vi "SECoP-getStoredCommand_2.vi"(8 "error in (no error)":errorcluster, 11 "DLL path (in)":T2) -> (0 "error out":errorcluster, 1 "arguments/setvalue":string, 2 "command/parameter path":string, 3 "DLL path (out)":T2, 4 "action":T1, 5 "command id":u64)   [LabVIEW 2023, in "SECoP.lvlib"]
doc: "Call <b>\"SECoP-getStoredCommand_2.vi\"</b> regulary to check, if there is something to do for any accessible. If yes, it will return successfully with an id, what to do, a parameter/command name and new set value or argument as JSON string.\n\n<b>DLL path</b> input and output of cluster from \"SECoP-Initialize.vi\"\n<b>command id</b> on match: command id for \"SECoP-putCommandAnswer_2.vi\"\n<b>action id</b> on match: action id to handle\n<b>command/parameter path</b> on match: full name of accessible\n<b>arguments/setvalue</b> on match with change or do: JSON input data from SECoP-client"
uses:
  SECoP.lvlib
  SECoP-libraries.ctl
  SECoP-action.ctl
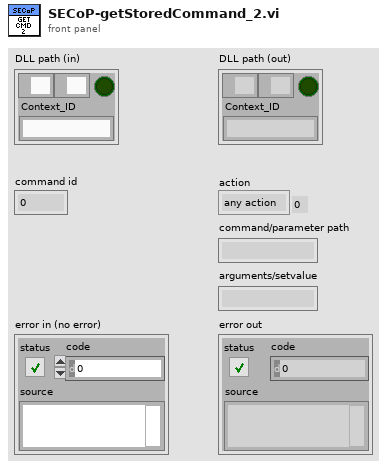
[diagram p1: front panel]
types:
  T1 = typedef "SECoP.lvlib/SECoP-action.ctl" = enum32{"any action", "read", "change", "do cmd"}
  T2 = typedef "SECoP.lvlib/SECoP-libraries.ctl" = cluster{"serverDLL":path, "variantDLL":path, "cleanup_mode":bool, "Context_ID":string}
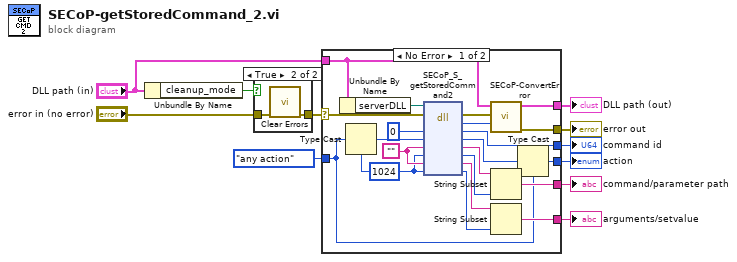
[diagram p0: block diagram]
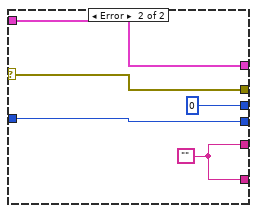
[diagram p3: hidden frame]
diagram:
  n1 = Unbundle By Name("DLL path (in)") -> ("cleanup_mode"=w6:bool)
  n2 = case shown="True" w6 {
    tunnel: "error in (no error)" -> [w12 w14]
    tunnel: [w12 w13] -> w4
    frame False {
    }
    frame True {
      n3 = call <vilib>:"Clear Errors.vi"("error in (no error)"=w14) -> ("error out"=w13:errorcluster)  [unwired: 5 in, 1 out]
    }
  }
  n4 = case shown="No Error" w4 {
    selector: w4 -> [w33 w39]
    tunnel: "DLL path (in)" -> [w15 w40]
    tunnel: [w34 w40] -> w11
    tunnel: [w35 w39] -> w10
    tunnel: [w24 u64 0 ("id")] -> w9
    tunnel: [w20 w36] -> w2
    tunnel: [w22 w37] -> w8
    tunnel: [w21 w37] -> w7
    tunnel: SECoP-action."any action" ("SECoP_action") -> [w19 w36]
    frame No Error {
      w18 = 1024 ("parameter size")
      w29 = ""
      n5 = Unbundle By Name(w15) -> ("serverDLL"=w16:path)
      n6 = Type Cast(type=w18, x=w19) -> (*(type *) &x=w17:i32)
      n7 = dll-call lib="Z:/Praktische Aufgaben/SECoP-LabVIEW2015/32bit/SECoP32.dll" fn="SECoP_S_getStoredCommand2"(path in=w16, error in=w33, "id"=u64 0, "command"=w17, "parameter"=w29, "parameter size"=w18, "value"=w29, "value size"=w18) -> (error out=w32:errorcluster, "return type"=w31:i32, "id"=w24:u64, "command"=w23:i32, "parameter"=w25:string, "parameter size"=w26:i32, "value"=w28:string, "value size"=w27:i32)  [unwired: 1 in, 1 out]
      n8 = call "SECoP-ConvertError.vi"("return code"=w31, "error in (no error)"=w32, "DLL path (in)"=w15) -> ("error out"=w35:errorcluster, "DLL path (out)"=w34:T2)  [unwired: 7 in]
      n9 = String Subset(string=w25, length (rest)=w26) -> (substring=w22:string)  [unwired: 1 in]
      n10 = String Subset(string=w28, length (rest)=w27) -> (substring=w21:string)  [unwired: 1 in]
      n11 = Type Cast(type=w19, x=w23) -> (*(type *) &x=w20:T1)
    }
    frame Error {
      w37 = ""
    }
  }
  "DLL path (out)" <- w11
  "error out" <- w10
  "command/parameter path" <- w8
  "command id" <- w9
  "arguments/setvalue" <- w7
  "action" <- w2
